vi "Listener.vi"(11 "Log Sinks":refnum<class "Log Sinks.lvclass">) -> ()   [LabVIEW 2019, in "TSC Event Logger.lvlib" / "Log Sinks.lvclass"]
doc: "A parallel sink loop that will be launched and housed as a location to receive logging packets. This is a private VI because it is not meant to be used outside the scope of the Log Sinks class.\n\n<b>Code Developed By:</b>\nTechnology Service Corporation\nBloomington, IN 47403\nwww.tsc.com/atcs\n\nDeveloper:\nDaniel Coons"
uses:
  Log Sinks.lvclass
  Log Sinks.lvclass/Log Sinks.ctl
  Log Data.ctl
  Log/Event Level.ctl
  TSC Event Logger.lvlib
panel:
  out "msg":string
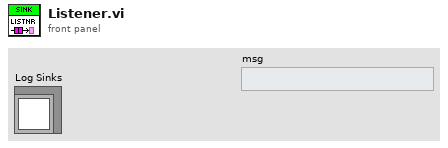
[diagram p1: front panel]
types:
  T1 = typedef "TSC Event Logger.lvlib/Log Data.ctl" = cluster{"Time":timestamp, "Level":T2, "Logger":string, "Message":string, "Arguments":string[]}
  T2 = typedef "TSC Event Logger.lvlib/Event Level.ctl" = enum16{"OFF", "TRACE", "DEBUG", "INFO", "WARN", "ERROR", "FATAL"}
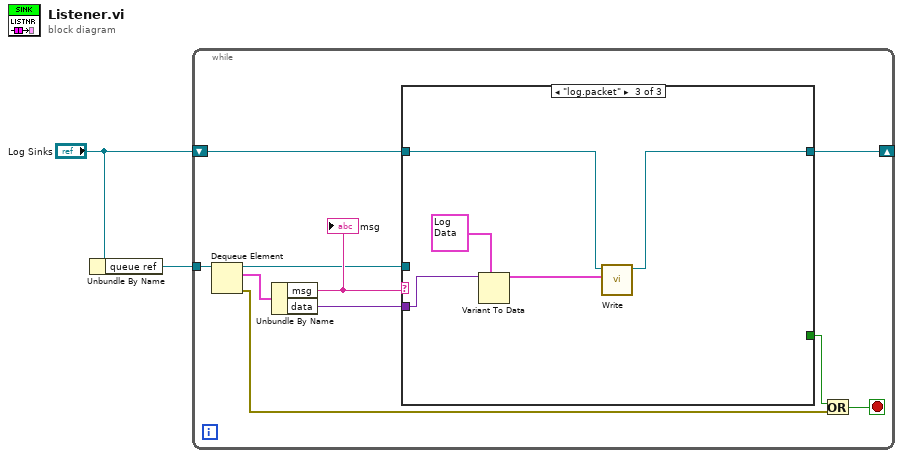
[diagram p0: block diagram]
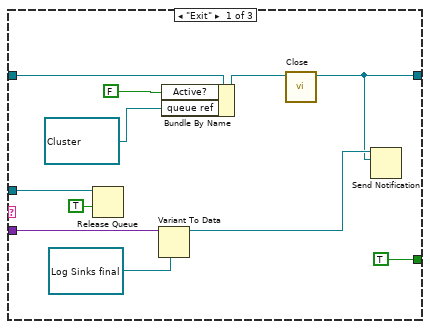
[diagram p2: hidden frame]
diagram:
  n1 = Unbundle By Name("Log Sinks") -> ("queue ref"=w1:refnum<queue>)
  n2 = while {
    tunnel: w1 -> [w12]
    shift-right: [w6] -> _
    shift-left: "Log Sinks" -> [w7]
    stop <- w4 stop-if-true
    n3 = Dequeue Element(queue=w12) -> (queue out=w8:refnum<queue>, element=w11:cluster{"msg":string, "data":variant}, error out=w3:errorcluster)  [unwired: 2 in, 1 out]
    n4 = Unbundle By Name(w11) -> ("msg"=w10:string, "data"=w9:variant)
    "msg" <- w10
    n5 = case shown="\"log.packet\"" w10 {
      tunnel: w9 -> [w16 _ w29]
      tunnel: [TRUE _ _] -> w5
      tunnel: w8 -> [w22 _ _]
      tunnel: w7 -> [w20 w24 w27]
      tunnel: [w13 w24 w26] -> w6
      frame "Exit" {
        n6 = Release Queue(queue=w22, force destroy? (F)=TRUE) -> ()  [unwired: 1 in, 3 out]
        n7 = Variant To Data(type=refnum<notifier> refnum ("notifier out"), Variant=w16) -> (data=w14:refnum<notifier>)  [unwired: 1 in, 1 out]
        n8 = Bundle By Name(cluster=w20, "Active?"=FALSE, "queue ref"=refnum<queue> refnum) -> (w17:refnum<class "Log Sinks.lvclass">)
        n9 = call-dynamic "Close.vi"("Log Sinks in"=w17) -> ("Log Sinks out"=w13:refnum<class "Log Sinks.lvclass">)  [unwired: 9 in, 1 out]
        n10 = Send Notification(notification=w13, notifier=w14) -> ()  [unwired: 1 in, 2 out]
      }
      frame Default {
      }
      frame "log.packet" {
        n11 = Variant To Data(type=T1 {"Time"=timestamp(0 s since 1904-01-01), "Level"=enum."INFO", "Logger"="", "Message"="", "Arguments"=[]} ("Log Data"), Variant=w29) -> (data=w25:T1)  [unwired: 1 in, 1 out]
        n12 = call-dynamic "Write.vi"("Log Data"=w25, "Log Sinks in"=w27) -> ("Log Sinks out"=w26:refnum<class "Log Sinks.lvclass">)  [unwired: 8 in, 1 out]
      }
    }
    n13 = Or(x=w5, y=w3) -> (x .or. y?=w4:bool)
  }
